vi "dateString.vi"() -> (3 "dateOUT":string)   [LabVIEW 2011]
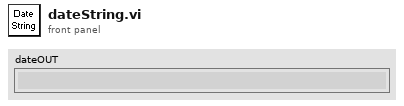
[diagram p1: front panel]
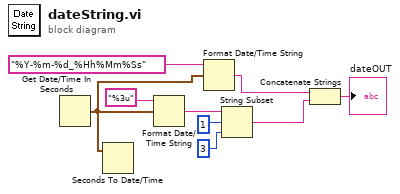
[diagram p0: block diagram]
diagram:
  n1 = Get Date/Time In Seconds() -> (seconds since 1Jan1904=w9:timestamp)
  n2 = Seconds To Date/Time(time stamp (now)=w9) -> ()  [unwired: 2 out]
  n3 = Format Date/Time String(time format string (%c)="%3u", seconds (now)=w9) -> (date/time string=w8:string)  [unwired: 1 out]
  n4 = Format Date/Time String(time format string (%c)="%Y-%m-%d_%Hh%Mm%Ss", seconds (now)=w9) -> (date/time string=w3:string)  [unwired: 1 out]
  n5 = String Subset(string=w8, offset (0)=1, length (rest)=3 ("length (rest)")) -> (substring=w2:string)
  n6 = Concatenate Strings(w3, w2) -> (→"dateOUT":string)
